vi "Measure Data to 2D Format All Plots.vi"(8 "error in":errorcluster, 11 "Graph Combined Reference":refnum<vi>) -> (0 "error out":errorcluster, 2 "2D String Data":string[][](array[string]), 3 "Graph Combined Reference":refnum<vi>, 5 "Title":string[](array[string]))   [LabVIEW 2023]
doc: "Use this VI to extract plot data and convert it to a table format."
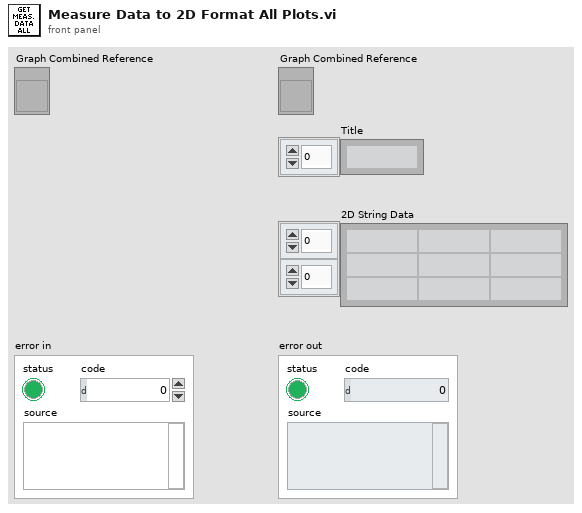
[diagram p1: front panel]
types:
  T1 = cluster{"Load currents":dbl[], "Efficiency":dbl[]}[]
  T2 = cluster{"Load currents":dbl[], "Efficiency":dbl[]}
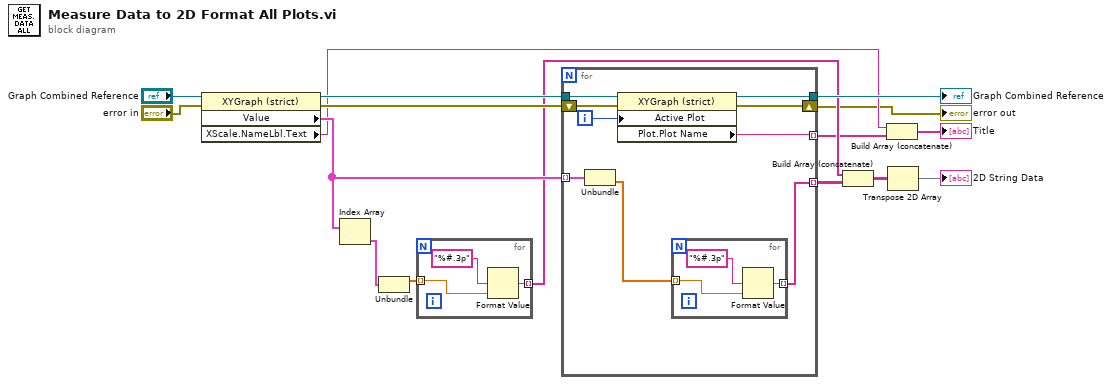
[diagram p0: block diagram]
diagram:
  n1 = property on="Property Node" class="XYGraph (strict)"(reference="Graph Combined Reference", error in="error in") -> (reference out=w14:refnum<vi>, error out=w13:errorcluster, "Value"=w10:T1, "XScale.NameLbl.Text"=w4:string)
  n2 = Index Array(array=w10) -> (element=w9:T2)  [unwired: 1 in]
  n3 = Unbundle(w9) -> ("Load currents"=w8:dbl[])  [unwired: 1 out]
  n4 = for {
    tunnel: [w19] -> w7 mode=indexing
    tunnel: w8 -> [w17] mode=indexing
    n5 = Format Value(format string="%#.3p", value (0)=w17) -> (output string=w19:string)  [unwired: 1 in]
  }
  n6 = for {
    tunnel: [w20] -> w11 mode=indexing
    tunnel: w10 -> [w28] mode=indexing
    tunnel: [w26] -> w6 mode=indexing
    tunnel: w14 -> [w25]
    tunnel: [w24] -> w12
    shift-right: [w22] -> w2
    shift-left: w13 -> [w23]
    i -> [w27]
    n7 = Unbundle(w28) -> ("Efficiency"=w21:dbl[])  [unwired: 1 out]
    n8 = property on="Property Node" class="XYGraph (strict)"(reference=w25, error in=w23, "Active Plot"=w27) -> (reference out=w24:refnum<vi>, error out=w22:errorcluster, "Plot.Plot Name"=w26:string)
    n9 = for {
      tunnel: [w31] -> w20 mode=indexing
      tunnel: w21 -> [w29] mode=indexing
      n10 = Format Value(format string="%#.3p", value (0)=w29) -> (output string=w31:string)  [unwired: 1 in]
    }
  }
  "Graph Combined Reference" <- w12
  "error out" <- w2
  n11 = Build Array (concatenate)(w7, w11) -> (w15:string[][])
  n12 = Build Array (concatenate)(w4, w6) -> (→"Title":string[])
  n13 = Transpose 2D Array(2D array=w15) -> (transposed array=→"2D String Data":string[][])
